vi "global_ui_stream_and_variable_connections.vi"() -> ()   [LabVIEW 2015]
uses:
  support_vis/message_queue/message_cluster.ctl
  type_definitions/variable_references.ctl
  support_vis/message_queue/message_queue.lvlib
panel:
  in  "Variable References":T1 caption="变量引用"
  in  "UI Stream Reader":refnum<k21> caption="UI网络流读取方端点"
  in  "UI Stream Writer":refnum<k21> caption="UI网络流写入方端点"
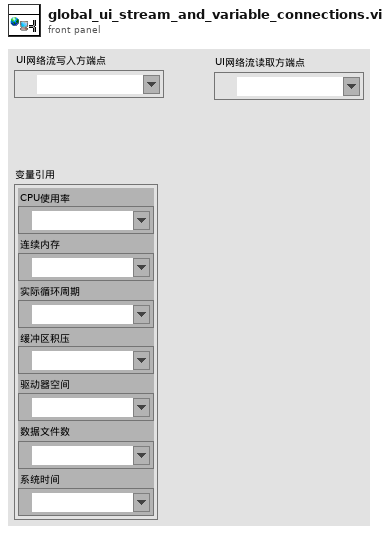
[diagram p1: front panel]
types:
  T1 = typedef "variable_references.ctl" = cluster{"CPU 1 Usage":refnum<k21>, "Free Memory":refnum<k21>, "Actual Loop Period":refnum<k21>, "CPU 2 Usage":refnum<k21>, "Drive Space":refnum<k21>, "Number of Data Files":refnum<k21>, "System Time":refnum<k21>}
diagram:
